vi "Get Pixels.vi"(8 "error in (no error)":errorcluster, 11 "Image in":refnum<class "Image.lvclass">) -> (0 "error out":errorcluster, 2 "Pixels":refnum<class "Pixel.lvclass">[][](array[class]), 3 "Image out":refnum<class "Image.lvclass">)   [LabVIEW 2020, in "RPI.SenseHat.Display.lvlib" / "Image.lvclass"]
doc: "Returns the image pixel array.\n\nNote: Pixels is the 2D array of Pixel."
uses:
  Image.lvclass
  Pixel/Pixel.lvclass
  Image.lvclass/Image.ctl
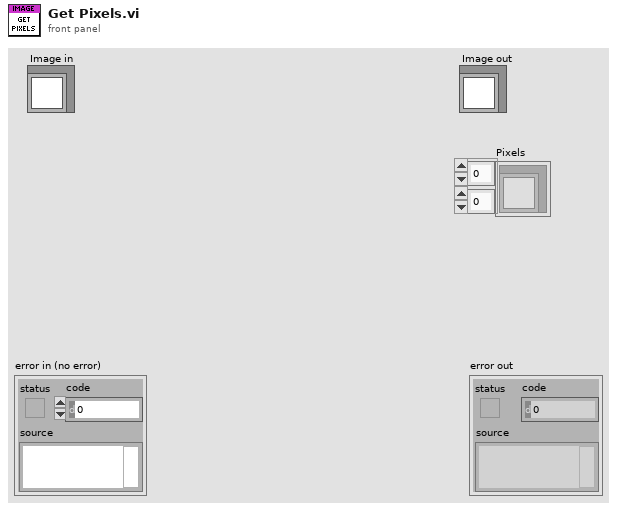
[diagram p1: front panel]
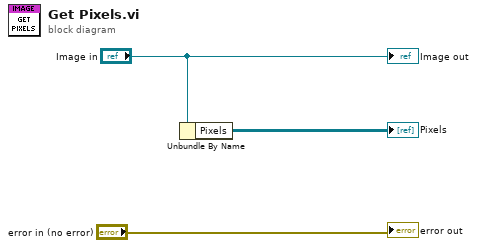
[diagram p0: block diagram]
diagram:
  n1 = Unbundle By Name("Image in") -> ("Pixels"=→"Pixels":refnum<class "Pixel.lvclass">[][])
  "error out" <- "error in (no error)"
  "Image out" <- "Image in"
